vi "Comdel CX.vi"() -> ()   [LabVIEW 2015]
doc: "Example VI that demonstrates all library features."
uses:
  PL Comdel CX.lvclass
panel:
  in  "disable rf":bool
  in  "enable rf":bool
  out "status":T1
  in  "serial watchdog time, s":u16
  in  "ramp-down time, s":dbl=0.1
  in  "ramp-up time, s":dbl=0.1
  in  "power, W":u16
  out "reflected power, W":u16
  out "forward power, W":u16
  in  "stop bits":u16(ring)=10 items=["1.0"=10, "1.5"=15, "2.0"=20]
  in  "parity":u16(ring) items=["None", "Odd", "Even", "Mark", "Space"]
  in  "data bits":u16=8
  out "Comdel":refnum<class "PL Comdel CX.lvclass">
  in  "baud rate":u32=9600
  in  "port":refnum<visa-resource-name>
  out "error":errorcluster
  in  "stop":bool
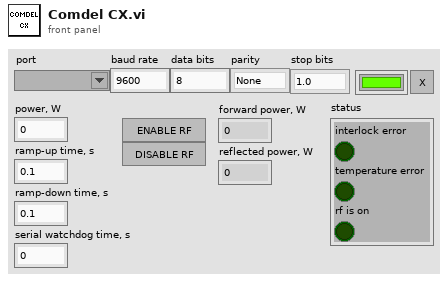
[diagram p1: front panel]
types:
  T1 = cluster{"interlock error":bool, "temperature error":bool, "rf is on":bool}
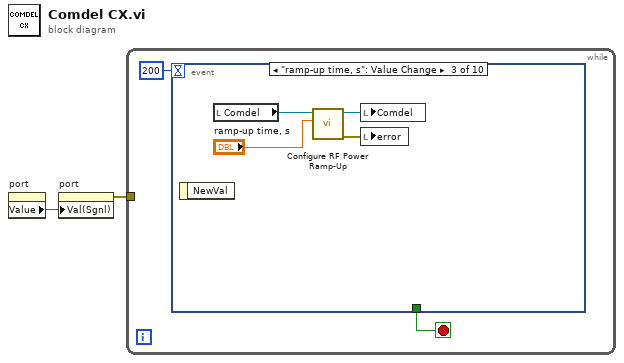
[diagram p0: block diagram]
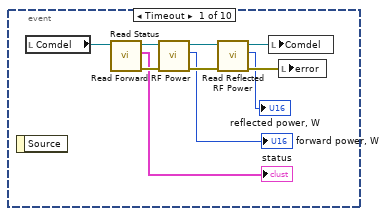
[diagram p2: hidden frame]
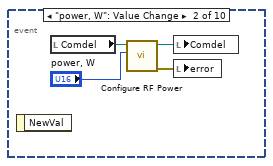
[diagram p3: hidden frame]
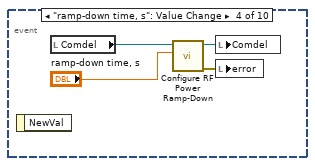
[diagram p4: hidden frame]
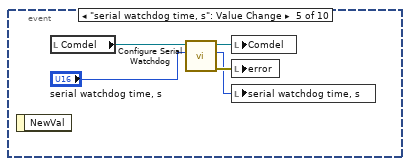
[diagram p5: hidden frame]
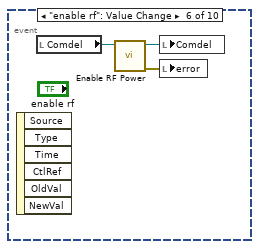
[diagram p6: hidden frame]
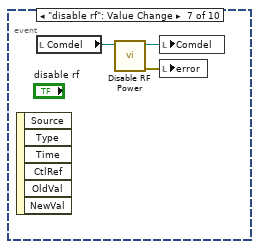
[diagram p7: hidden frame]
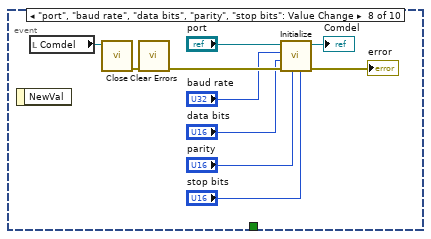
[diagram p8: hidden frame]
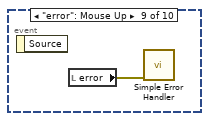
[diagram p9: hidden frame]
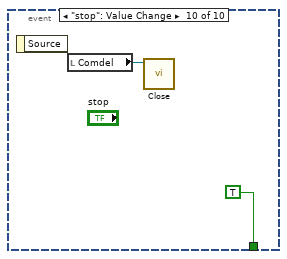
[diagram p10: hidden frame]
diagram:
  n1 = property on="port" class="VISAName"() -> ("Value"=w1:refnum<visa-resource-name>)  [unwired: 2 in, 2 out]
  n2 = property on="port" class="VISAName"("Val(Sgnl)"=w1) -> (error out=w2:errorcluster)  [unwired: 2 in, 1 out]
  n3 = while {
    tunnel: w2 -> [_]
    stop <- w3 stop-if-true
    n4 = event shown="[2] \"ramp-up time, s\": Value Change" {
      selector: _ -> [_ _ _ _ _ _ _ _ _ _]
      dyn-events: _ -> [_ _ _ _ _ _ _ _ _ _]
      timeout: 200 -> [_ _ _ _ _ _ _ _ _ _]
      tunnel: [_ _ _ _ _ _ _ _ _ TRUE ("stop")] -> w3
      event Timeout {
        n5 = event-data() -> ()  [unwired: 1 in, 1 out]
        n6 = local read "Comdel"() -> (w8:refnum<class "PL Comdel CX.lvclass">)
        n7 = call "Read Status.vi"("Comdel in"=w8) -> ("error out"=w6:errorcluster, "status"=→"status":T1, "Comdel out"=w7:refnum<class "PL Comdel CX.lvclass">)  [unwired: 8 in]
        n8 = call "Read Forward RF Power.vi"("error in (no error)"=w6, "Comdel in"=w7) -> ("error out"=w11:errorcluster, "power, W"=→"forward power, W":u16, "Comdel out"=w14:refnum<class "PL Comdel CX.lvclass">)  [unwired: 7 in]
        n9 = call "Read Reflected RF Power.vi"("error in (no error)"=w11, "Comdel in"=w14) -> ("error out"=w12:errorcluster, "power, W"=→"reflected power, W":u16, "Comdel out"=w13:refnum<class "PL Comdel CX.lvclass">)  [unwired: 7 in]
        n10 = local write "Comdel"(w13) -> ()
        n11 = local write "error"(w12) -> ()
      }
      event "power, W": Value Change {
        n12 = event-data() -> ()  [unwired: 1 in, 1 out]
        n13 = local read "Comdel"() -> (w18:refnum<class "PL Comdel CX.lvclass">)
        n14 = call "Configure RF Power.vi"("power, W"="power, W", "Comdel in"=w18) -> ("error out"=w16:errorcluster, "Comdel out"=w17:refnum<class "PL Comdel CX.lvclass">)  [unwired: 8 in]
        n15 = local write "Comdel"(w17) -> ()
        n16 = local write "error"(w16) -> ()
      }
      event "ramp-up time, s": Value Change {
        n17 = event-data() -> ()  [unwired: 1 in, 1 out]
        n18 = local read "Comdel"() -> (w21:refnum<class "PL Comdel CX.lvclass">)
        n19 = call "Configure RF Power Ramp-Up.vi"("time, s"="ramp-up time, s", "Comdel in"=w21) -> ("error out"=w20:errorcluster, "Comdel out"=w22:refnum<class "PL Comdel CX.lvclass">)  [unwired: 8 in]
        n20 = local write "Comdel"(w22) -> ()
        n21 = local write "error"(w20) -> ()
      }
      event "ramp-down time, s": Value Change {
        n22 = event-data() -> ()  [unwired: 1 in, 1 out]
        n23 = local read "Comdel"() -> (w23:refnum<class "PL Comdel CX.lvclass">)
        n24 = call "Configure RF Power Ramp-Down.vi"("time, s"="ramp-down time, s", "Comdel in"=w23) -> ("error out"=w26:errorcluster, "Comdel out"=w25:refnum<class "PL Comdel CX.lvclass">)  [unwired: 8 in]
        n25 = local write "Comdel"(w25) -> ()
        n26 = local write "error"(w26) -> ()
      }
      event "serial watchdog time, s": Value Change {
        n27 = event-data() -> ()  [unwired: 1 in, 1 out]
        n28 = local read "Comdel"() -> (w31:refnum<class "PL Comdel CX.lvclass">)
        n29 = call "Configure Serial Watchdog.vi"("time, s (0 = disabled)"="serial watchdog time, s", "Comdel in"=w31) -> ("error out"=w29:errorcluster, "time, s"=w27:u16, "Comdel out"=w30:refnum<class "PL Comdel CX.lvclass">)  [unwired: 7 in]
        n30 = local write "Comdel"(w30) -> ()
        n31 = local write "error"(w29) -> ()
        n32 = local write "serial watchdog time, s"(w27) -> ()
      }
      event "enable rf": Value Change {
        n33 = event-data() -> ()  [unwired: 1 in, 6 out]
        n34 = local read "Comdel"() -> (w34:refnum<class "PL Comdel CX.lvclass">)
        n35 = call "Enable RF Power.vi"("Comdel in"=w34) -> ("error out"=w32:errorcluster, "Comdel out"=w33:refnum<class "PL Comdel CX.lvclass">)  [unwired: 9 in]
        n36 = local write "Comdel"(w33) -> ()
        n37 = local write "error"(w32) -> ()
      }
      event "disable rf": Value Change {
        n38 = event-data() -> ()  [unwired: 1 in, 6 out]
        n39 = local read "Comdel"() -> (w36:refnum<class "PL Comdel CX.lvclass">)
        n40 = call "Disable RF Power.vi"("Comdel in"=w36) -> ("error out"=w35:errorcluster, "Comdel out"=w37:refnum<class "PL Comdel CX.lvclass">)  [unwired: 9 in]
        n41 = local write "Comdel"(w37) -> ()
        n42 = local write "error"(w35) -> ()
      }
      event "port", "baud rate", "data bits", "parity", "stop bits": Value Change {
        n43 = event-data() -> ()  [unwired: 1 in, 1 out]
        n44 = local read "Comdel"() -> (w47:refnum<class "PL Comdel CX.lvclass">)
        n45 = call "Close.vi"("Comdel in"=w47) -> ("error out"=w38:errorcluster)  [unwired: 10 in]
        n46 = call <vilib>:"Clear Errors.vi"("error in (no error)"=w38) -> ("error out"=w43:errorcluster)  [unwired: 5 in, 1 out]
        n47 = call "Initialize.vi"("stop bits (1.0)"="stop bits", "parity (none)"="parity", "error in (no error)"=w43, "data bits (8)"="data bits", "baud rate (9600)"="baud rate", "port"="port") -> ("error out"=→"error":errorcluster, "Comdel out"=→"Comdel":refnum<class "PL Comdel CX.lvclass">)  [unwired: 4 in]
      }
      event "error": Mouse Up {
        n48 = event-data() -> ()  [unwired: 1 in, 1 out]
        n49 = local read "error"() -> (w48:errorcluster)
        n50 = call <vilib>:"Simple Error Handler.vi"("error in (no error)"=w48) -> ()  [unwired: 4 in, 5 out]
      }
      event "stop": Value Change {
        n51 = event-data() -> ()  [unwired: 1 in, 1 out]
        n52 = local read "Comdel"() -> (w49:refnum<class "PL Comdel CX.lvclass">)
        n53 = call "Close.vi"("Comdel in"=w49) -> ()  [unwired: 10 in, 1 out]
      }
    }
  }
